vi "VirtualBench_Set_Voltage.vi"(8 "Error In":errorcluster, 9 "Voltage level":dbl, 10 "VB Power Supply Output Channel":tag="ps/+25V" caption="Channel", 11 "VB Device Name":tag="VirtualBench" caption="Device Name") -> (0 "Error Out":errorcluster)   [LabVIEW 2016]
uses:
  <vilib>/VirtualBench/_PS Configure Voltage Output0.vi
  <vilib>/VirtualBench/VirtualBench.lvlib
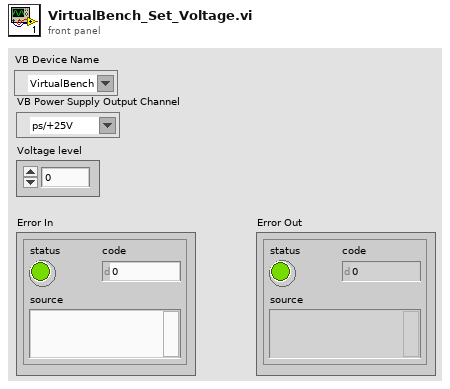
[diagram p1: front panel]
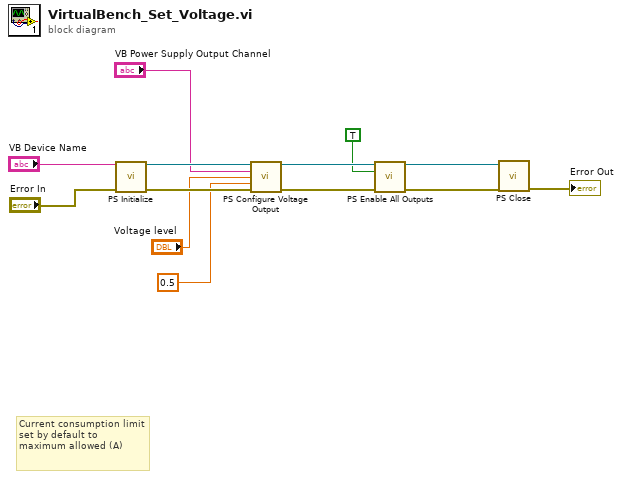
[diagram p0: block diagram]
diagram:
  # "Current consumption limit set by default to maximum allowed (A)"
  n1 = call <vilib>:"PS Initialize.vi"("Device Name"="VB Device Name", "Error In"="Error In") -> ("Instrument Handle Out"=w11:refnum<k21>, "Error Out"=w13:errorcluster)  [unwired: 12 in]
  n2 = call-poly <vilib>:"PS Configure Voltage Output.vi"("Instrument Handle In"=w11, "Channel"="VB Power Supply Output Channel", "Voltage Level"="Voltage level", "Current Limit"=0.5, "Error In"=w13) -> ("Instrument Handle Out"=w7:refnum<k21>, "Error Out"=w6:errorcluster)  [unwired: 9 in]
  n3 = call <vilib>:"PS Enable All Outputs.vi"("Instrument Handle In"=w7, "Enable Outputs"=TRUE, "Error In"=w6) -> ("Instrument Handle Out"=w4:refnum<k21>, "Error Out"=w3:errorcluster)  [unwired: 11 in]
  n4 = call <vilib>:"PS Close.vi"("Instrument Handle In"=w4, "Error In"=w3) -> ("Error Out"=→"Error Out":errorcluster)  [unwired: 13 in]
